vi "ReplaceClassControls.vi"(6 "ClassPath":path, 8 "error in (no error)":errorcluster, 9 "properties":T1, 11 "vi refnum":refnum<vi>) -> (0 "error out":errorcluster, 3 "ClassLibref":refnum<vi>)   [LabVIEW 2013, in "GenLVOOP.lvclass"]
uses:
  GenLVOOP.lvclass
  baseClass/propertyDef.ctl
  baseClass/types.ctl
  baseClass/baseClass.lvclass
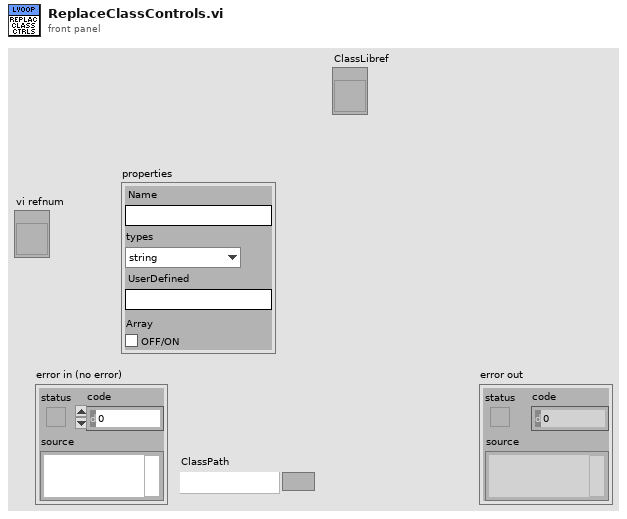
[diagram p1: front panel]
types:
  T1 = typedef "baseClass.lvclass/propertyDef.ctl" = cluster{"Name":string, "types":T2, "UserDefined":string, "Array":bool}
  T2 = typedef "baseClass.lvclass/types.ctl" = enum16{"string", "int", "decimal", "bool", "class", "enum"}
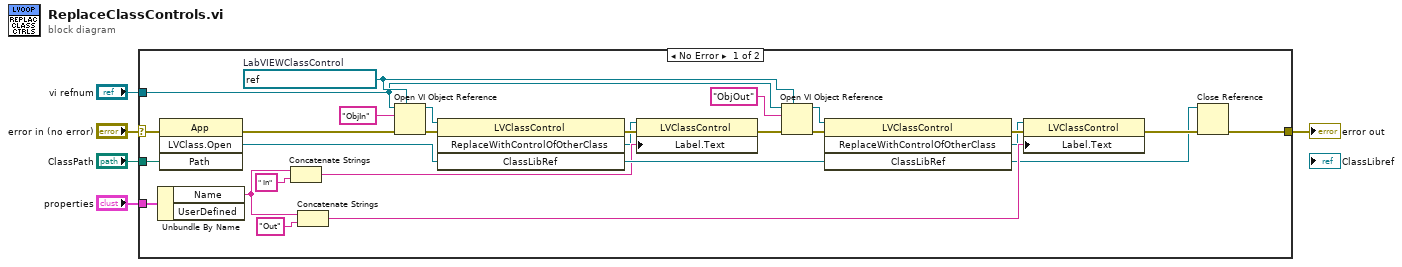
[diagram p0: block diagram]
diagram:
  n1 = case shown="No Error" "error in (no error)" {
    selector: "error in (no error)" -> [w12 w33]
    tunnel: [w7 w33] -> w4
    tunnel: "properties" -> [w32 _]
    tunnel: "ClassPath" -> [w29 _]
    tunnel: "vi refnum" -> [w21 _]
    frame No Error {
      w26 = refnum<vi> refnum  # LabVIEWClassControl
      n2 = Unbundle By Name(w32) -> ("Name"=w15:string)  [unwired: 1 out]
      n3 = invoke class="App" method="LVClass.Open"(error in=w12, "Path"=w29) -> (error out=w11:errorcluster, "LVClass.Open"=w28:refnum<vi>)  [unwired: 2 in, 2 out]
      n4 = Concatenate Strings(w15, " In" ("string")) -> (w18:string)
      n5 = Concatenate Strings(w15, "Out" ("string")) -> (w13:string)
      n6 = Open VI Object Reference(7:w26, 8:w11, 10:"ObjIn" ("name/order"), 11:w21) -> (0:w27:errorcluster, 3:w30:refnum<vi>)
      n7 = invoke class="LVClassControl" method="ReplaceWithControlOfOtherClass"(reference=w30, error in=w27, "ClassLibRef"=w28) -> (error out=w20:errorcluster, "ReplaceWithControlOfOtherClass"=w9:refnum<vi>, "ClassLibRef"=w22:refnum<vi>)  [unwired: 1 in, 1 out]
      n8 = property class="LVClassControl"(reference=w9, error in=w20, "Label.Text"=w18) -> (error out=w17:errorcluster)  [unwired: 1 out]
      n9 = Open VI Object Reference(7:w26, 8:w17, 10:"ObjOut" ("name/order"), 11:w21) -> (0:w23:errorcluster, 3:w24:refnum<vi>)
      n10 = invoke class="LVClassControl" method="ReplaceWithControlOfOtherClass"(reference=w24, error in=w23, "ClassLibRef"=w22) -> (error out=w16:errorcluster, "ReplaceWithControlOfOtherClass"=w8:refnum<vi>, "ClassLibRef"=w6:refnum<vi>)  [unwired: 1 in, 1 out]
      n11 = property class="LVClassControl"(reference=w8, error in=w16, "Label.Text"=w13) -> (error out=w10:errorcluster)  [unwired: 1 out]
      n12 = Close Reference(reference=w6, error in (no error)=w10) -> (error out=w7:errorcluster)
    }
    frame Error {
    }
  }
  "error out" <- w4
